vi "Mobility-Vt Calculator_Saturation_12_09_10a_JW.vi"(0 "Vg Column":dbl[](array[numeric]), 1 "Dielectric Constant":dbl, 5 "Sat Id Column":dbl[](array[numeric]), 7 "NumPts":dbl=5.0, 9 "Length":dbl, 11 "Width":dbl, 12 "Dielectric Thickness":dbl) -> (2 "Check Cluster":T1, 3 "Log Graph":cluster{dbl[], dbl[]}[](graph), 4 "Mobility-Sat":dbl format="%#_4e", 6 "VT-Sat":dbl, 8 "Index-Sat":dbl, 10 "Sqrt Plot":cluster{dbl[], dbl[]}[](graph), 13 "Raw Graph":cluster{dbl[], dbl[]}[](graph), 14 "Off I-Sat":dbl format="%_6g", 15 "On/Off I-Sat":dbl)   [LabVIEW 2012]
uses:
  <vilib>/Analysis/NI_AALPro.lvlib
panel:
  out "Off I-Sat 2":dbl
  out "Capacitance (C)":dbl
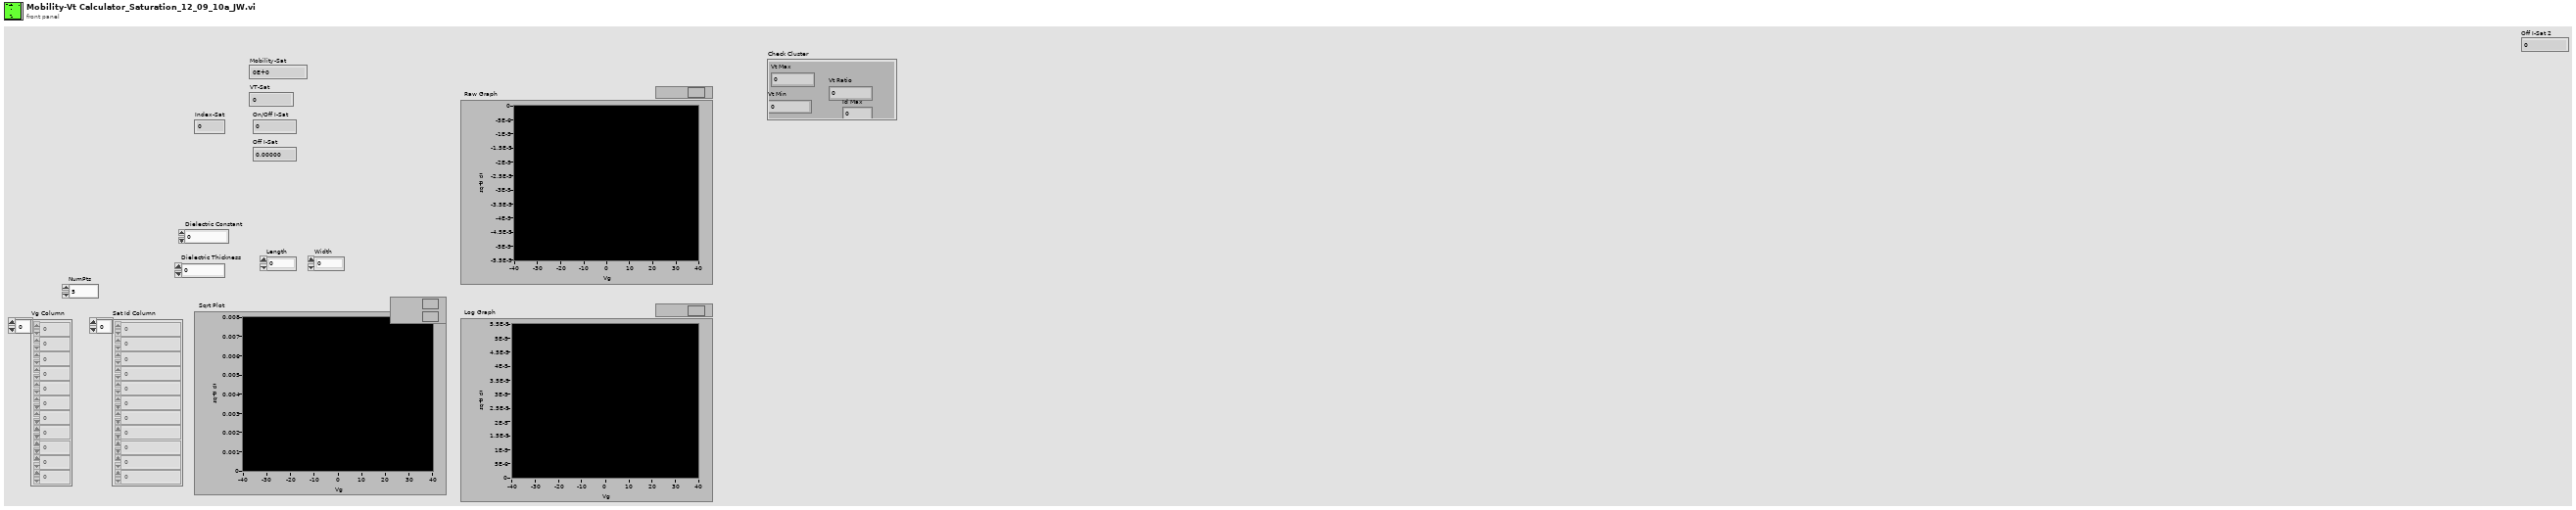
[diagram p1: front panel]
types:
  T1 = cluster{"Vt Max":dbl, "Vt Min":dbl, "Vt Ratio":dbl, "Id Max":dbl}
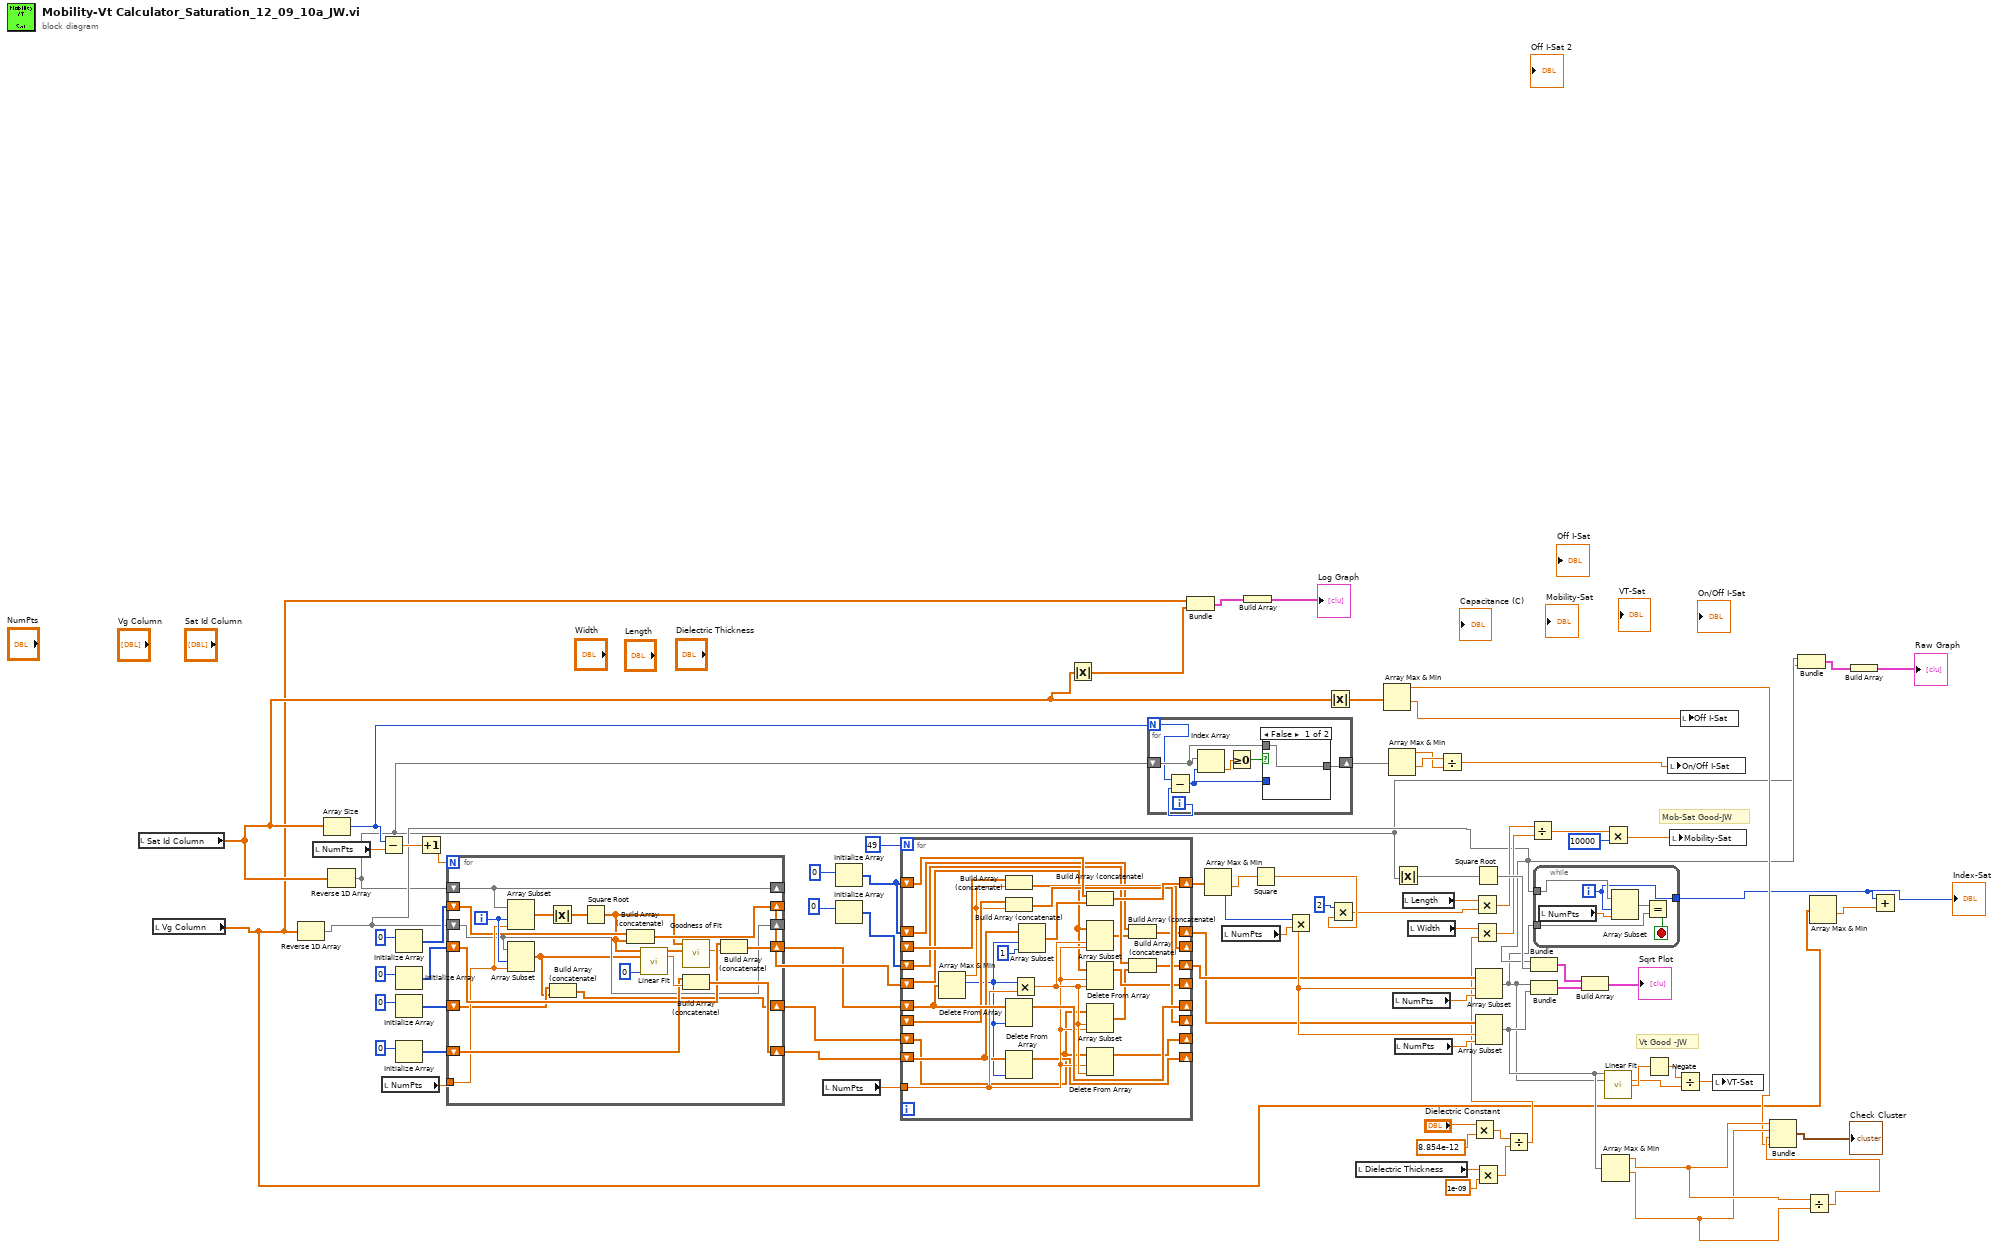
[diagram p0: block diagram]
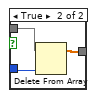
[diagram p2: hidden frame]
diagram:
  # "Mob-Sat Good-JW"
  # "Vt Good -JW"
  n1 = local read "Sat Id Column"() -> (w8:dbl[])
  n2 = local read "Vg Column"() -> (w4:dbl[])
  n3 = Reverse 1D Array(array=w4) -> (reversed array=w11:dbl[])
  n4 = local read "NumPts"() -> (w77:dbl)
  n5 = Array Size(array=w8) -> (size(s)=w23:i32)
  n6 = Reverse 1D Array(array=w8) -> (reversed array=w9:dbl[])
  n7 = Subtract(x=w23, y=w77) -> (x-y=w74:dbl)
  n8 = local read "NumPts"() -> (w80:dbl)
  n9 = Initialize Array(0) -> (w61:i32[])  [unwired: 1 in]
  n10 = Initialize Array(0) -> (w50:i32[])  [unwired: 1 in]
  n11 = Initialize Array(0) -> (w62:i32[])  [unwired: 1 in]
  n12 = Initialize Array(0) -> (w49:i32[])  [unwired: 1 in]
  n13 = Increment(x=w74) -> (x+1=w75:dbl)
  n14 = for {
    N: w75 -> [_]
    shift-right: [w87] -> _
    shift-left: w11 -> [w87]
    shift-right: [w96] -> _
    shift-left: w9 -> [w96]
    shift-right: [w100] -> w55
    shift-left: w49 -> [w99]
    shift-right: [w98] -> w57
    shift-left: w50 -> [w97]
    tunnel: w80 -> [w92]
    shift-right: [w90] -> w63
    shift-left: w61 -> [w91]
    shift-right: [w88] -> w64
    shift-left: w62 -> [w89]
    i -> [w102]
    n15 = Array Subset(array=w96, index=w102, length=w92) -> (w95:dbl[])
    n16 = Array Subset(array=w87, index=w102, length=w92) -> (w86:dbl[])
    n17 = Absolute Value(x=w95) -> (abs(x)=w94:dbl[])
    n18 = Build Array (concatenate)(w89, w86) -> (w88:dbl[])
    n19 = Square Root(x=w94) -> (sqrt(x)=w83:dbl[])
    n20 = Build Array (concatenate)(w91, w83) -> (w90:dbl[])
    n21 = call <vilib>:"Linear Fit.vi"("Y"=w83, "X"=w86, "method"=0) -> ("Best Linear Fit"=w85:dbl[], "slope"=w101:dbl)  [unwired: 8 in, 3 out]
    n22 = call <vilib>:"Goodness of Fit.vi"("Best Fit"=w85, "Y"=w83) -> ("R-square"=w84:dbl)  [unwired: 6 in, 3 out]
    n23 = Build Array (concatenate)(w99, w101) -> (w100:dbl[])
    n24 = Build Array (concatenate)(w97, w84) -> (w98:dbl[])
  }
  n25 = local read "NumPts"() -> (w76:dbl)
  n26 = Initialize Array(0) -> (w70:i32[])  [unwired: 1 in]
  n27 = Initialize Array(0) -> (w65:i32[])  [unwired: 1 in]
  n28 = for {
    N: 49 -> [_]
    shift-right: [w127] -> _
    shift-left: w57 -> [w128]
    shift-right: [w107] -> _
    shift-left: w55 -> [w108]
    shift-right: [w124] -> w56
    shift-left: w70 -> [w123]
    shift-right: [w122] -> _
    shift-left: _ -> [w121]
    shift-right: [w120] -> _
    shift-left: _ -> [w119]
    shift-right: [w118] -> _
    shift-left: w63 -> [w104]
    shift-right: [w116] -> _
    shift-left: w64 -> [w103]
    tunnel: w76 -> [w115]
    shift-right: [w114] -> w67
    shift-left: w70 -> [w113]
    shift-right: [w112] -> w68
    shift-left: w65 -> [w111]
    n29 = Array Max & Min(array=w128) -> (max value=w106:dbl, max index (indices)=w105:i32)  [unwired: 2 out]
    n30 = Build Array (concatenate)(w119, w106) -> (w120:dbl[])
    n31 = Build Array (concatenate)(w121, w106) -> (w122:dbl[])
    n32 = Delete From Array(array=w128, index=w105) -> (array with subset deleted=w127:dbl[])  [unwired: 1 in, 1 out]
    n33 = Delete From Array(array=w108, index=w105) -> (array with subset deleted=w107:dbl[])  [unwired: 1 in, 1 out]
    n34 = Multiply(x=w105, y=w115) -> (x*y=w117:dbl)
    n35 = Array Subset(array=w108, index=w105, length=1) -> (w125:dbl[])
    n36 = Build Array (concatenate)(w123, w125) -> (w124:dbl[])
    n37 = Array Subset(array=w104, index=w117, length=w115) -> (w109:dbl[])
    n38 = Delete From Array(array=w104, length=w115, index=w117) -> (array with subset deleted=w118:dbl[])  [unwired: 1 out]
    n39 = Array Subset(array=w103, index=w117, length=w115) -> (w110:dbl[])
    n40 = Delete From Array(array=w103, length=w115, index=w117) -> (array with subset deleted=w116:dbl[])  [unwired: 1 out]
    n41 = Build Array (concatenate)(w113, w109) -> (w114:dbl[])
    n42 = Build Array (concatenate)(w111, w110) -> (w112:dbl[])
  }
  n43 = Absolute Value(x=w8) -> (abs(x)=w7:dbl[])
  n44 = for {
    N: w23 -> [w131]
    shift-right: [w134] -> w27
    shift-left: w9 -> [w135]
    i -> [w130]
    n45 = Subtract(x=w131, y=w130) -> (x-y=w129:i32)
    n46 = Index Array(array=w135, index=w129) -> (element=w132:dbl)
    n47 = Greater Or Equal To 0?(x=w132) -> (x >= 0?=w133:bool)
    n48 = case shown="False" w133 {
      tunnel: w135 -> [w136 w139]
      tunnel: w129 -> [_ w137]
      tunnel: [w136 w138] -> w134
      frame False {
      }
      frame True {
        n49 = Delete From Array(array=w139, index=w137) -> (array with subset deleted=w138:dbl[])  [unwired: 1 in, 1 out]
      }
    }
  }
  n50 = Bundle("Vg Column"=w4, w7) -> (w6:cluster{"Vg Column":dbl[], dbl[]})  [unwired: 1 in]
  n51 = Array Max & Min(array=w56) -> (min value=w53:dbl, min index (indices)=w69:i32)  [unwired: 2 out]
  n52 = local read "NumPts"() -> (w79:dbl)
  n53 = Build Array(w6) -> (→"Log Graph":cluster{"Vg Column":dbl[], dbl[]}[])
  n54 = Square(x=w53) -> (x^2=w48:dbl)
  n55 = Multiply(x=w69, y=w79) -> (x*y=w71:dbl)
  n56 = Absolute Value(x=w8) -> (abs(x)=w22:dbl[])
  n57 = Multiply(x=2, y=w48) -> (x*y=w47:dbl)
  n58 = local read "Dielectric Thickness"() -> (w33:dbl)
  n59 = Array Max & Min(array=w22) -> (max value=w15:dbl, min value=w21:dbl)  [unwired: 2 out]
  n60 = Array Max & Min(array=w27) -> (max value=w25:dbl, min value=w26:dbl)  [unwired: 2 out]
  n61 = local read "NumPts"() -> (w78:dbl)
  n62 = Absolute Value(x=w9) -> (abs(x)=w59:dbl[])
  n63 = local read "NumPts"() -> (w81:dbl)
  n64 = local read "Length"() -> (w36:dbl)
  n65 = local read "Width"() -> (w37:dbl)
  n66 = Divide(x=w26, y=w25) -> (x/y=w24:dbl)
  n67 = Multiply(x="Dielectric Constant", y=8.854e-12) -> (x*y=w29:dbl)
  n68 = Multiply(x=w36, y=w47) -> (x*y=w46:dbl)
  n69 = Square Root(x=w59) -> (sqrt(x)=w73:dbl[])
  n70 = Multiply(x=w33, y=1e-09) -> (x*y=w31:dbl)
  n71 = Array Subset(array=w68, index=w71, length=w78) -> (w10:dbl[])
  n72 = Array Subset(array=w67, index=w71, length=w81) -> (w20:dbl[])
  n73 = Divide(x=w29, y=w31) -> (x/y=w28:dbl)
  n74 = Multiply(x=w37, y=w28) -> (x*y=w45:dbl)
  n75 = Divide(x=w46, y=w45) -> (x/y=w43:dbl)
  n76 = Bundle(w11, w73) -> (w14:cluster{dbl[], dbl[]})  [unwired: 1 in]
  n77 = Bundle(w10, w20) -> (w72:cluster{dbl[], dbl[]})  [unwired: 1 in]
  n78 = while {
    tunnel: w11 -> [w144]
    tunnel: w10 -> [w140]
    tunnel: [w141] -> w2
    i -> [w141]
    stop <- w145 stop-if-true
    n79 = local read "NumPts"() -> (w142:dbl)
    n80 = Array Subset(array=w144, index=w141, length=w142) -> (w143:dbl[])
    n81 = Equal?(x=w143, y=w140) -> (x = y?=w145:bool)
  }
  "Index-Sat" <- w2
  n82 = Build Array(w14, w72) -> (→"Sqrt Plot":cluster{dbl[], dbl[]}[])
  n83 = Array Max & Min(array=w20) -> (max value=w19:dbl, min value=w18:dbl)  [unwired: 2 out]
  n84 = Multiply(x=w43, y=10000) -> (x*y=w35:dbl)
  n85 = call <vilib>:"Linear Fit.vi"("Y"=w20, "X"=w10) -> ("slope"=w39:dbl, "intercept"=w41:dbl)  [unwired: 9 in, 3 out]
  n86 = Negate(x=w41) -> (-x=w40:dbl)
  n87 = local write "On/Off I-Sat"(w24) -> ()
  n88 = local write "Mobility-Sat"(w35) -> ()
  n89 = Divide(x=w40, y=w39) -> (x/y=w34:dbl)
  n90 = local write "Off I-Sat"(w21) -> ()
  n91 = local write "VT-Sat"(w34) -> ()
  n92 = Bundle(w11, w9) -> (w13:cluster{dbl[], dbl[]})  [unwired: 1 in]
  n93 = Divide(x=w19, y=w18) -> (x/y=w17:dbl)
  n94 = Bundle(w19, w18, w17, w15) -> (→"Check Cluster":cluster{dbl, dbl, dbl, dbl})  [unwired: 1 in]
  n95 = Array Max & Min(array=w4) -> (min value=w3:dbl)  [unwired: 3 out]
  n96 = Build Array(w13) -> (→"Raw Graph":cluster{dbl[], dbl[]}[])
  n97 = Add(x=w2, y=w3) -> ()  [unwired: 1 out]
